vi "notifier2.vi"() -> ()   [LabVIEW 2013]
panel:
  in  "Run":bool
  out "LED 2":bool
  out "LED 1":bool
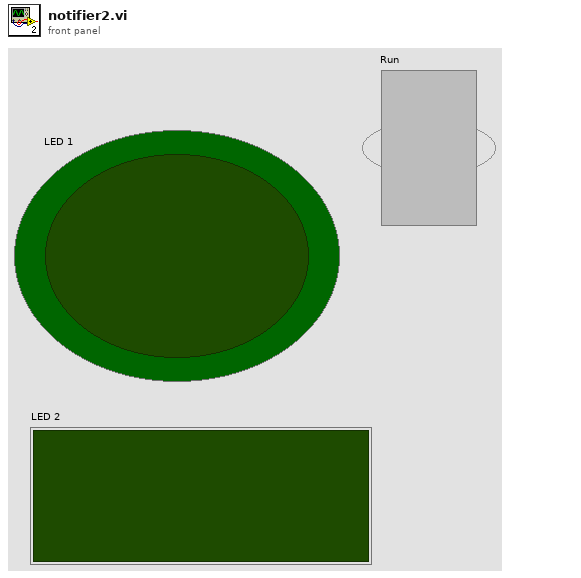
[diagram p1: front panel]
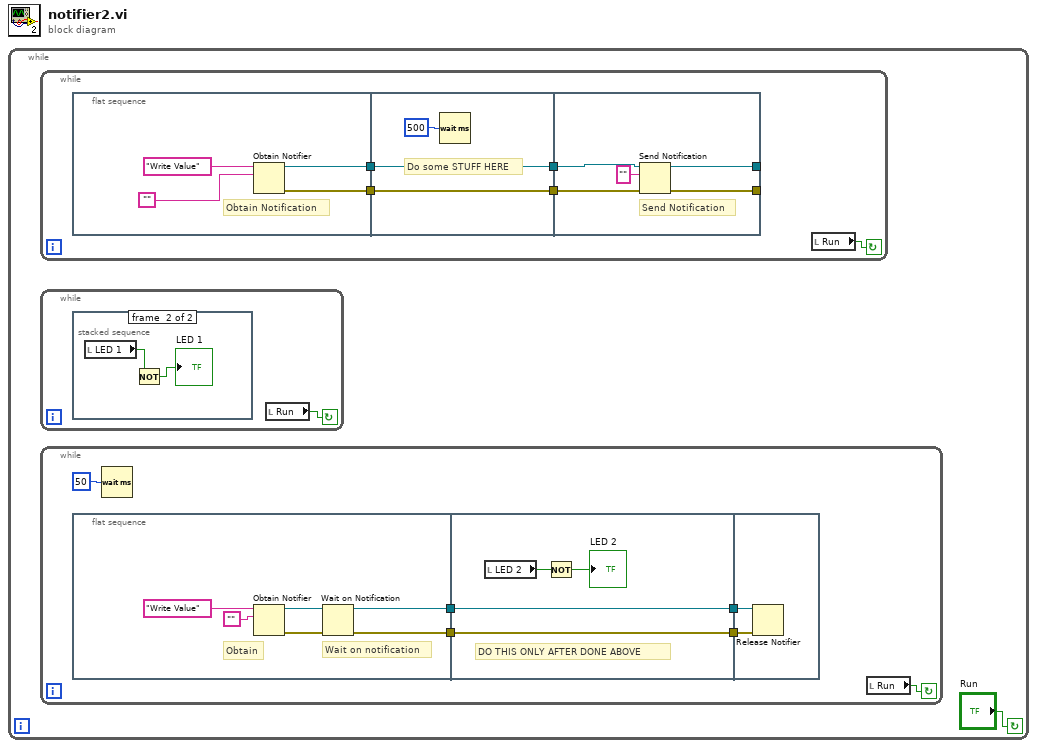
[diagram p0: block diagram]
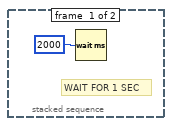
[diagram p2: hidden frame]
diagram:
  n1 = while {
    stop <- "Run" continue-if-true
    n2 = while {
      stop <- w28 continue-if-true
      n3 = flat-sequence {
        tunnel: [w31] -> w27
        tunnel: [w30] -> w26
        tunnel: w27 -> [w34]
        tunnel: w26 -> [w33]
        tunnel: [w34] -> w25
        tunnel: [w33] -> w24
        tunnel: w25 -> [w40]
        tunnel: [w39] -> _
        tunnel: w24 -> [w38]
        tunnel: [w37] -> _
        frame #0 {
          # "Obtain Notification"
          n4 = Obtain Notifier(name (unnamed)="Write Value", notification data type="") -> (notifier out=w31:refnum<notifier>, error out=w30:errorcluster)  [unwired: 2 in, 1 out]
        }
        frame #1 {
          # "Do some STUFF HERE"
          n5 = Wait (ms)(milliseconds to wait=u32 500) -> ()  [unwired: 1 out]
        }
        frame #2 {
          # "Send Notification"
          n6 = Send Notification(notification="", notifier=w40, error in (no error)=w38) -> (notifier out=w39:refnum<notifier>, error out=w37:errorcluster)
        }
      }
      n7 = local read "Run"() -> (w28:bool)
    }
    n8 = while {
      stop <- w20 continue-if-true
      n9 = stacked-sequence {
        frame #0 {
          # "WAIT FOR 1 SEC"
          n10 = Wait (ms)(milliseconds to wait=u32 2000) -> ()  [unwired: 1 out]
        }
        frame #1 {
          n11 = local read "LED 1"() -> (w23:bool)
          n12 = Not(x=w23) -> (.not. x?=→"LED 1":bool)
        }
      }
      n13 = local read "Run"() -> (w20:bool)
    }
    n14 = while {
      stop <- w7 continue-if-true
      n15 = flat-sequence {
        tunnel: [w9] -> w5
        tunnel: [w8] -> w4
        tunnel: w5 -> [w15]
        tunnel: w4 -> [w14]
        tunnel: [w15] -> w3
        tunnel: [w14] -> w2
        tunnel: w3 -> [w19]
        tunnel: w2 -> [w18]
        frame #0 {
          # "Wait on notification"
          # "Obtain"
          n16 = Obtain Notifier(name (unnamed)="Write Value", notification data type="") -> (notifier out=w11:refnum<notifier>, error out=w10:errorcluster)  [unwired: 2 in, 1 out]
          n17 = Wait on Notification(notifier=w11, error in (no error)=w10) -> (notifier out=w9:refnum<notifier>, error out=w8:errorcluster)  [unwired: 2 in, 2 out]
        }
        frame #1 {
          # "DO THIS ONLY AFTER DONE ABOVE"
          n18 = local read "LED 2"() -> (w16:bool)
          n19 = Not(x=w16) -> (.not. x?=→"LED 2":bool)
        }
        frame #2 {
          n20 = Release Notifier(notifier=w19, error in (no error)=w18) -> ()  [unwired: 1 in, 3 out]
        }
      }
      n21 = Wait (ms)(milliseconds to wait=u32 50) -> ()  [unwired: 1 out]
      n22 = local read "Run"() -> (w7:bool)
    }
  }
